vi "Server Generate Event.vi"(8 "error in":errorcluster, 10 "event data":T1={"client request"={"meas config"={"fs [Hz]"=0.0, "count [smpl]"=0, "aperture [s]"=0.0, "trigger"={"source"=enum."Immediate", "level [V]"=0.0, "coupling"=enum."DC", "slope"=enum."POS"}, "ranges [Vpk]"=[], "QWTB parameters"=[]}, "mode"=enum."Raw", "processing setup"={"mode"=enum."Raw", "call after avgs?"=FALSE, "calculate?"=FALSE, "raw mode"={"command"="", "result mode"=enum."Display console output (only Octave)", "res variable"=""}, "QWTB"={"QWTB path"=path "", "alg filter path"="", "alg ids"=[], "alg parameters"=[], "parsed parameters"=[], "selected alg"=0, "selected unc mode"=enum."None", "qwtb mcc"=100, "qwtb timeout"=90, "qwtb covg"=95.0}}}, "GUI request"={"start"=FALSE, "setup"=FALSE, "setup&start"=FALSE}, "command"=enum."Identify"}, 11 "server event ref":refnum<vi>) -> (0 "error out":errorcluster)   [LabVIEW 2013]
doc: "Create server command."
uses:
  Server Event Start.ctl
  measure/Meas Sampling Configuration.ctl
  adc/ADC Trig Config.ctl
  adc/ADC Trig Mode Source.ctl
  adc/ADC Trig Coupling.ctl
  adc/ADC Trig Slope.ctl
  measure/processing/QWTB/Meas Proc QWTB Algorithm Parameter Data.ctl
  measure/processing/Meas Process Mode.ctl
  measure/processing/Meas Process Config.ctl
  measure/processing/Meas Process Raw Config.ctl
  measure/processing/Meas Process Raw Result Mode.ctl
  measure/processing/QWTB/Meas Proc QWTB Setup.ctl
  measure/processing/QWTB/Meas Proc QWTB Uncertainty Mode.ctl
  Server Event GUI command.ctl
  Server Event Command.ctl
  <vilib>/event_ctls.llb/usereventprio.ctl
  Server Event Ref.ctl
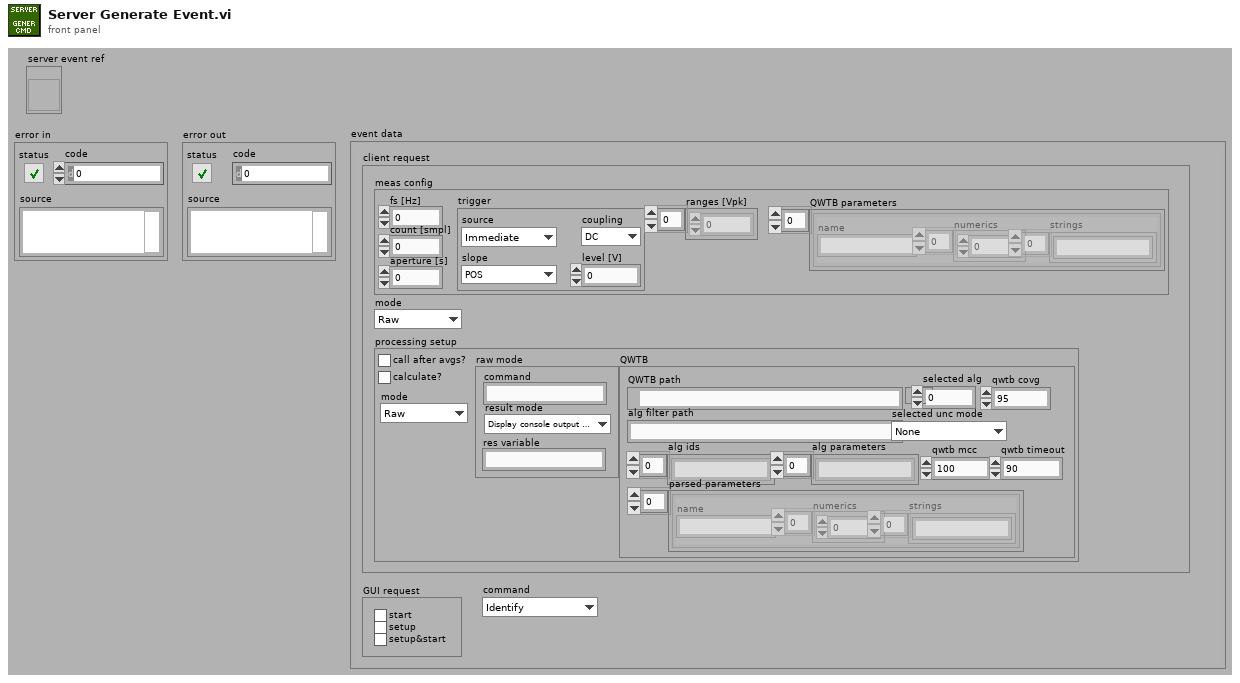
[diagram p1: front panel]
types:
  T1 = typedef "Server Event Start.ctl" = cluster{"client request":cluster{"meas config":T2, "mode":T8, "processing setup":T9}, "GUI request":T14, "command":T15}
  T2 = typedef "Meas Sampling Configuration.ctl" = cluster{"fs [Hz]":dbl, "count [smpl]":i64, "aperture [s]":dbl, "trigger":T3, "ranges [Vpk]":dbl[], "QWTB parameters":T7[]}
  T3 = typedef "ADC Trig Config.ctl" = cluster{"source":T4, "level [V]":dbl, "coupling":T5, "slope":T6}
  T4 = typedef "ADC Trig Mode Source.ctl" = enum16{"Immediate", "External", "Level"}
  T5 = typedef "ADC Trig Coupling.ctl" = enum16{"DC", "AC"}
  T6 = typedef "ADC Trig Slope.ctl" = enum16{"POS", "NEG"}
  T7 = typedef "Meas Proc QWTB Algorithm Parameter Data.ctl" = cluster{"name":string, "numerics":dbl[], "strings":string[]}
  T8 = typedef "Meas Process Mode.ctl" = enum16{"Raw", "QWTB"}
  T9 = typedef "Meas Process Config.ctl" = cluster{"mode":T8, "call after avgs?":bool, "calculate?":bool, "raw mode":T10, "QWTB":T12}
  T10 = typedef "Meas Process Raw Config.ctl" = cluster{"command":string, "result mode":T11, "res variable":string}
  T11 = typedef "Meas Process Raw Result Mode.ctl" = enum16{"Display console output (only Octave)", "Display string variable", "Display result file %respath%"}
  T12 = typedef "Meas Proc QWTB Setup.ctl" = cluster{"QWTB path":path, "alg filter path":string, "alg ids":string[], "alg parameters":string[], "parsed parameters":T7[], "selected alg":i32, "selected unc mode":T13, "qwtb mcc":i32, "qwtb timeout":i32, "qwtb covg":dbl}
  T13 = typedef "Meas Proc QWTB Uncertainty Mode.ctl" = enum16{"None", "GUF", "Monte Carlo"}
  T14 = typedef "Server Event GUI command.ctl" = cluster{"start":bool, "setup":bool, "setup&start":bool}
  T15 = typedef "Server Event Command.ctl" = enum16{"None", "Reset", "Identify", "Start", "Get status", "Get result"}
  T16 = typedef "Server Event Ref.ctl" = refnum<user-event>
  T17 = typedef "usereventprio.ctl" = enum32{"high priority", "normal priority"}
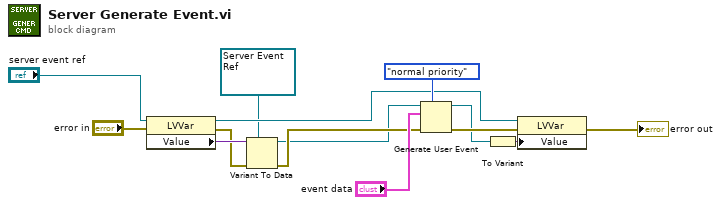
[diagram p0: block diagram]
diagram:
  n1 = property class="LVVar"(reference="server event ref", error in="error in") -> (reference out=w10:refnum<vi>, error out=w5:errorcluster, "Value"=w6:variant)
  n2 = Variant To Data(error in=w5, type=T16 refnum ("user event out"), Variant=w6) -> (data=w3:T16, error out=w4:errorcluster)
  n3 = Generate User Event(priority (normal)=usereventprio."normal priority", user event=w3, event data cluster="event data", error in=w4) -> (user event out=w9:T16, error out=w12:errorcluster)
  n4 = To Variant(anything=w9) -> (Variant=w7:variant)
  n5 = property class="LVVar"(reference=w10, error in=w12, "Value"=w7) -> (error out=→"error out":errorcluster)  [unwired: 1 out]
